vi "Not.vi"(1 "In":bool) -> (0 "Out":bool)   [LabVIEW 2012]
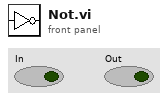
[diagram p1: front panel]
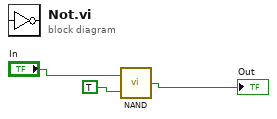
[diagram p0: block diagram]
diagram:
  n1 = call "NAND.vi"("b"=TRUE ("y"), "a"="In") -> ("x"=→"Out":bool)
